vi "Barcode Print.vi"(1 "part type":string, 2 "Manual?":bool, 4 "error in":errorcluster, 5 "Part History Number":string, 6 "Plant Number":u8 max=9, 7 "Customer Number":string, 8 "Color":string, 9 "Serial Number":string, 10 "Inalfa Part Number":string, 11 "Frame Barcode Formats":T1[](array[typedef])) -> (0 "error out":errorcluster)   [LabVIEW 2018]
uses:
  typedefs/barcode format params.ctl
  typedefs/barcode printer types.ctl
  typedefs/open tcp connections.ctl
  <vilib>/Instr/_visa.llb/VISA Configure Serial Port (Instr).vi
panel:
  out "concatenated string":string
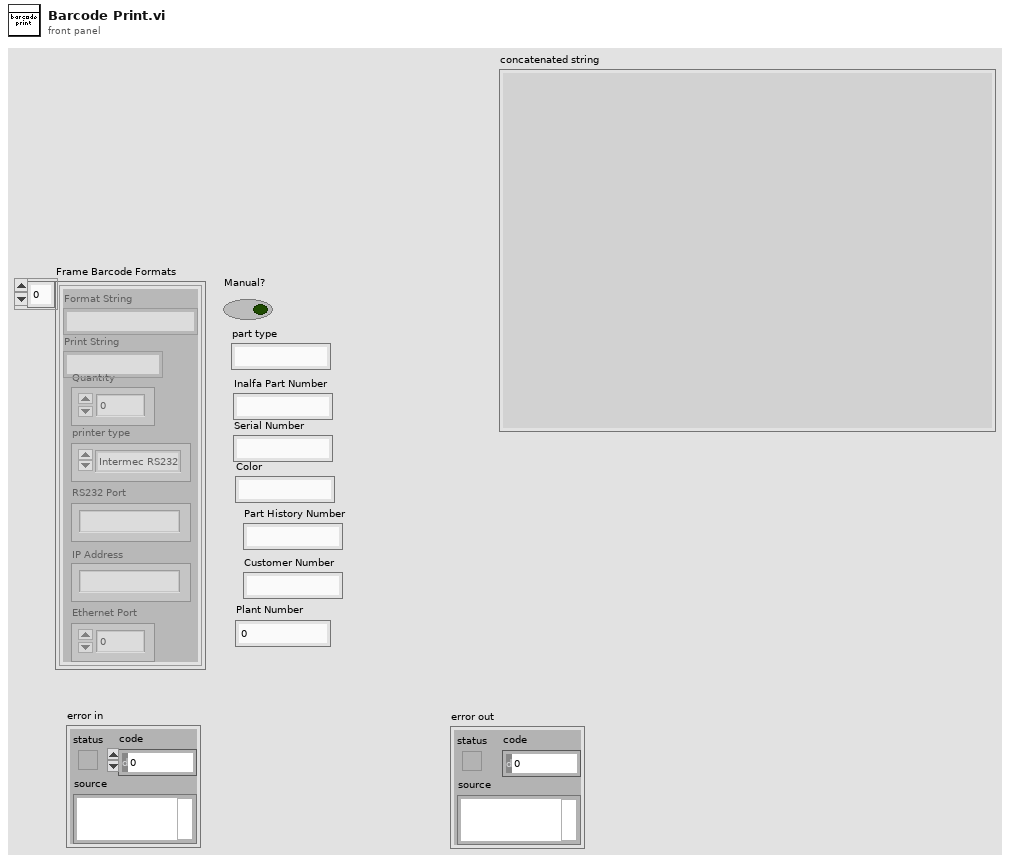
[diagram p1: front panel]
types:
  T1 = typedef "barcode format params.ctl" = cluster{"Format String":string, "Print String":string, "Quantity":u8, "printer type":T2, "RS232 Port":string, "IP Address":string, "Ethernet Port":u32}
  T2 = typedef "barcode printer types.ctl" = enum16{"Intermec RS232", "Intermec Ethernet"}
  T3 = typedef "open tcp connections.ctl" = cluster{"ip address":string, "connection ID":refnum<k5>}
  T4 = cluster{"Frame Barcode Formats":T1[], "VISA resource name":refnum<visa-resource-name>, "Format String":string, "Print String":string, "Inalfa Part Number":string, "Serial Number":string, "Color":string, "Customer Number":string, "Part History Number":string, "Plant Number":u8, "Manual?":bool, "part type":string, "to print":string[], "open rs232 ports":refnum<visa-resource-name>[], "open tcp ports":T3[]}
  T5 = typedef "imagedata.ctl" = cluster{"image type":i32, "image depth":i32, "image":u8[], "mask":u8[], "colors":u32[], "Rectangle":cluster{"left":i16, "top":i16, "right":i16, "bottom":i16}}
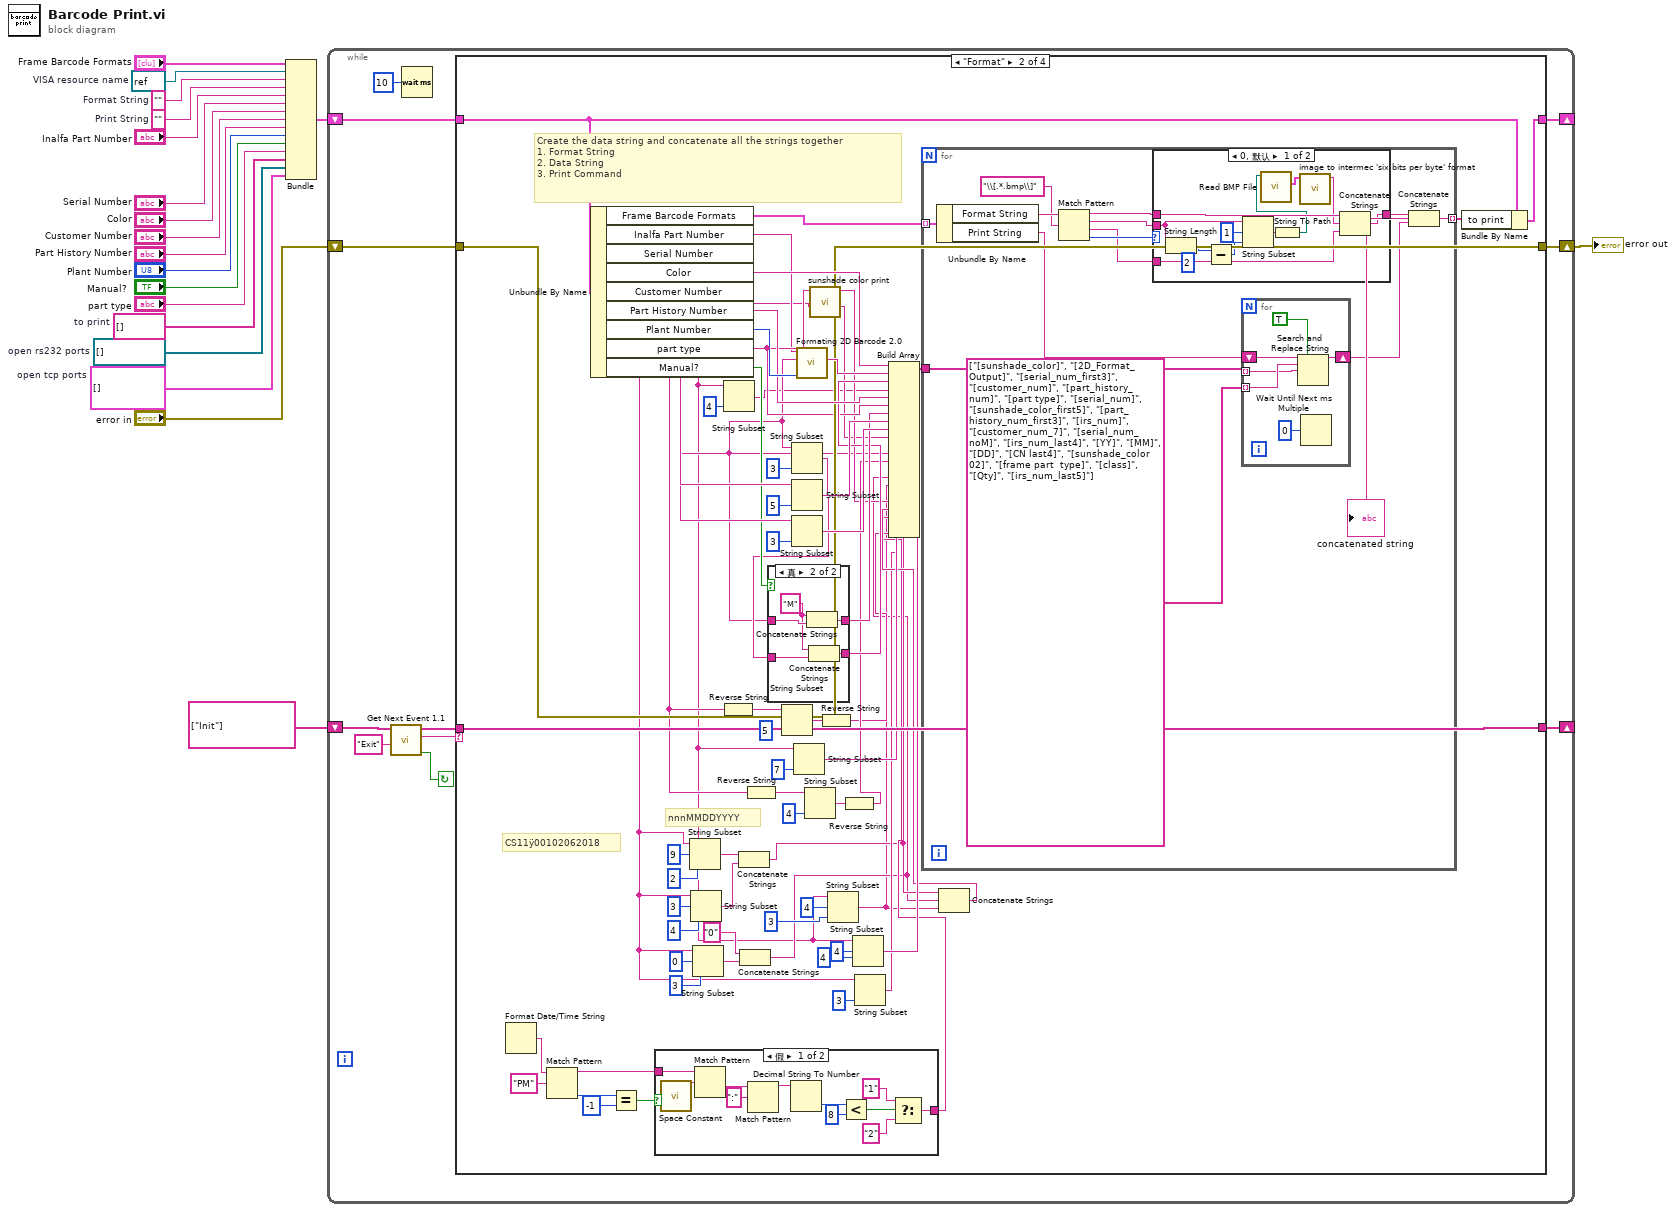
[diagram p0: block diagram]
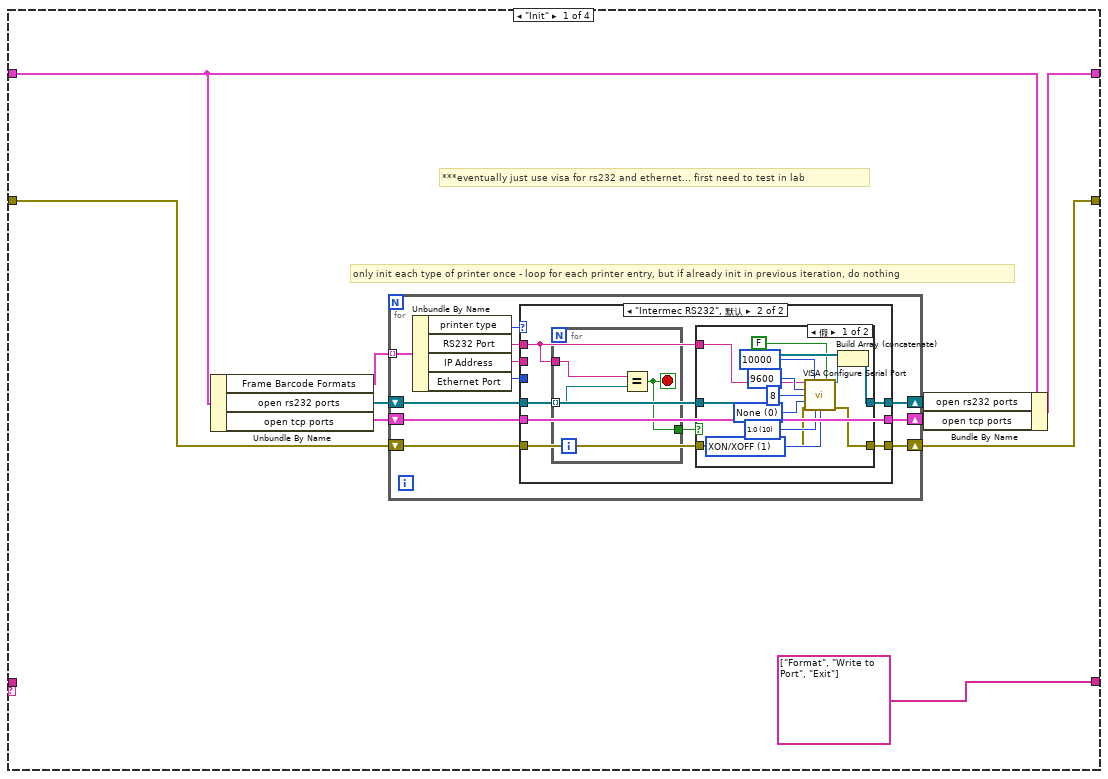
[diagram p2: hidden frame]
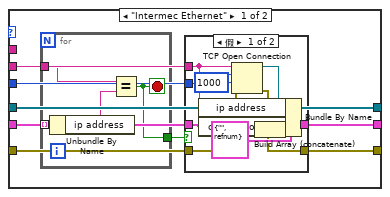
[diagram p3: hidden frame]
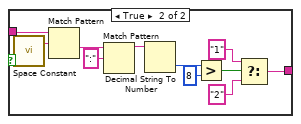
[diagram p6: hidden frame]
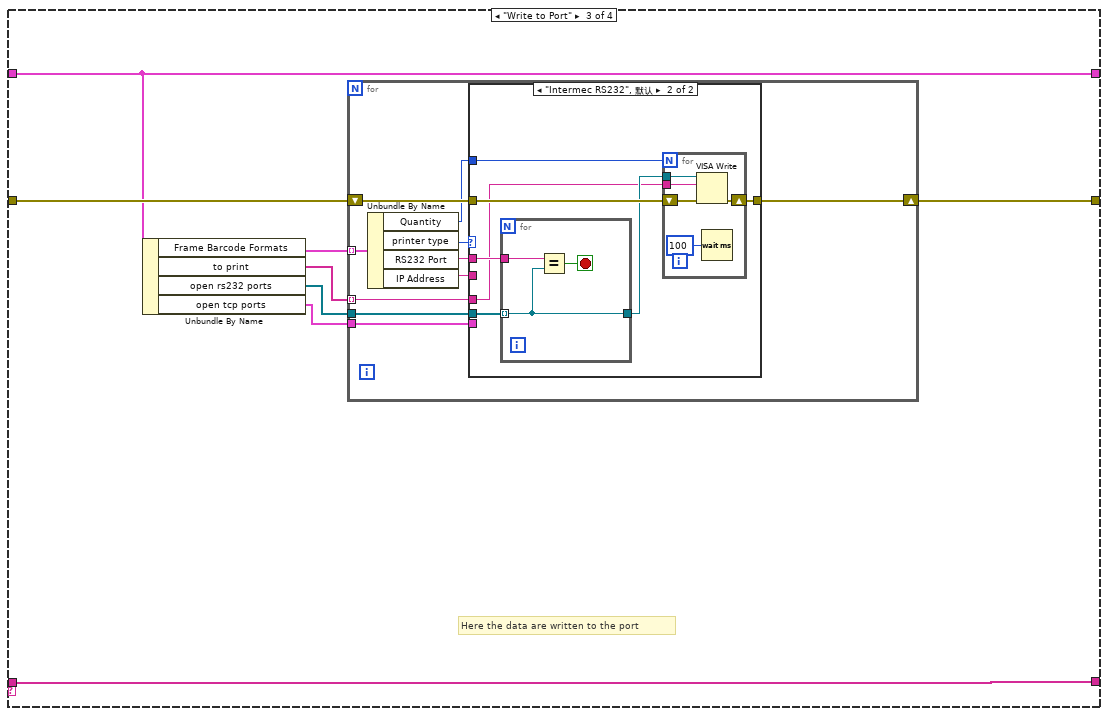
[diagram p9: hidden frame]
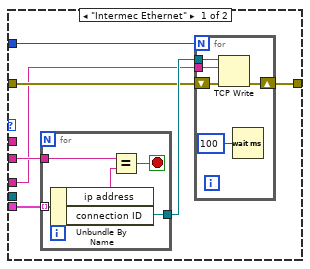
[diagram p10: hidden frame]
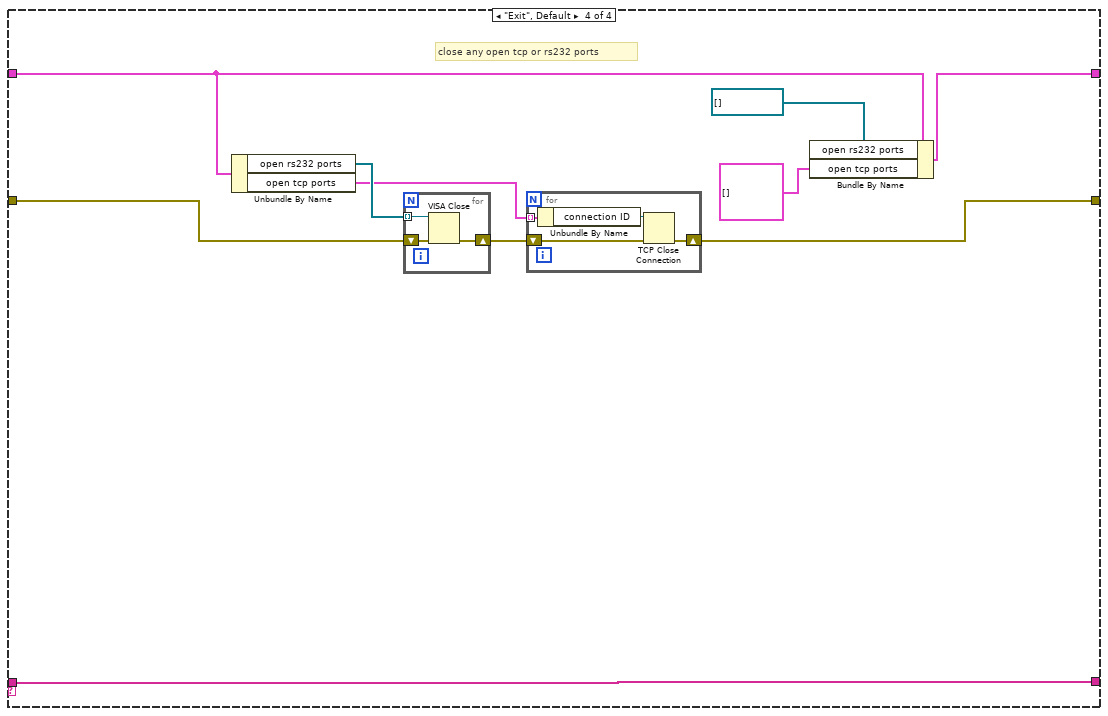
[diagram p11: hidden frame]
diagram:
  w1 = T3[] []  # open tcp ports
  w2 = refnum<visa-resource-name>[] []  # open rs232 ports
  w3 = string[] []  # to print
  w16 = ""  # Print String
  w17 = refnum<visa-resource-name> refnum  # VISA resource name
  w18 = ""  # Format String
  n1 = Bundle("Frame Barcode Formats"="Frame Barcode Formats", "VISA resource name"=w17, "Format String"=w18, "Print String"=w16, "Inalfa Part Number"="Inalfa Part Number", "Serial Number"="Serial Number", "Color"="Color", "Customer Number"="Customer Number", "Part History Number"="Part History Number", "Plant Number"="Plant Number", "Manual?"="Manual?", "part type"="part type", "to print"=w3, "open rs232 ports"=w2, "open tcp ports"=w1) -> (w19:T4)  [unwired: 1 in]
  n2 = while {
    shift-right: [w28] -> _
    shift-left: string[] ["Init"] ("Event queue out") -> [w27]
    shift-right: [w24] -> _
    shift-left: w19 -> [w25]
    shift-right: [w20] -> w4
    shift-left: "error in" -> [w21]
    stop <- w26 continue-if-true
    n3 = call "Get Next Event 1.1.vi"("Exit Event"="Exit", "event queue in"=w27) -> ("Condition (Exit:F)"=w26:bool, "next event"=w30:string, "event queue out"=w29:string[])  [unwired: 6 in, 1 out]
    n4 = Wait (ms)(milliseconds to wait=u32 10) -> ()  [unwired: 1 out]
    n5 = case shown="\"Format\"" w30 {
      tunnel: w29 -> [_ w148 w234 w286]
      tunnel: [string[] ["Format", "Write to Port", "Exit"] ("event queue out") w148 w234 w286] -> w28
      tunnel: w25 -> [w38 w166 w231 w281]
      tunnel: [w40 w165 w231 w280] -> w24
      tunnel: w21 -> [w35 w139 w233 w285]
      tunnel: [w34 w139 w232 w283] -> w20
      frame "Init" {
        # "***eventually just use visa for rs232 and ethernet... first need to test in lab"
        # "only init each type of printer once - loop for each printer entry, but if already init in previous iteration, do nothing"
        n6 = Unbundle By Name(w38) -> ("Frame Barcode Formats"=w33:T1[], "open rs232 ports"=w32:refnum<visa-resource-name>[], "open tcp ports"=w31:T3[])
        n7 = for {
          tunnel: w33 -> [w51] mode=indexing
          shift-right: [w45] -> w37
          shift-left: w32 -> [w47]
          shift-right: [w46] -> w36
          shift-left: w31 -> [w48]
          shift-right: [w41] -> w34
          shift-left: w35 -> [w49]
          n8 = Unbundle By Name(w51) -> ("printer type"=w50:T2, "RS232 Port"=w44:string, "IP Address"=w43:string, "Ethernet Port"=w42:u32)
          n9 = case shown="\"Intermec RS232\", 默认" w50 {
            tunnel: w49 -> [w53 w77]
            tunnel: w48 -> [w56 w81]
            tunnel: w47 -> [w59 w80]
            tunnel: [w57 w81] -> w46
            tunnel: [w59 w79] -> w45
            tunnel: w44 -> [_ w78]
            tunnel: w43 -> [w55 _]
            tunnel: w42 -> [w54 _]
            tunnel: [w52 w76] -> w41
            frame "Intermec Ethernet" {
              n10 = for {
                tunnel: w56 -> [w75] mode=indexing
                tunnel: w55 -> [w74]
                tunnel: [w72] -> w58
                stop <- w72 stop-if-true
                n11 = Unbundle By Name(w75) -> ("ip address"=w73:string)
                n12 = Equal?(x=w74, y=w73) -> (x = y?=w72:bool)
              }
              n13 = case shown="假" w58 {
                tunnel: [w66 w71] -> w57
                tunnel: w56 -> [w67 w71]
                tunnel: w55 -> [w63 _]
                tunnel: w54 -> [w69 _]
                tunnel: w53 -> [w61 w70]
                tunnel: [w60 w70] -> w52
                frame False {
                  n14 = TCP Open Connection(address=w63, remote port or service name=w69, timeout ms (60000)=1000, error in (no error)=w61) -> (connection ID=w62:refnum<k5>, error out=w60:errorcluster)  [unwired: 1 in]
                  n15 = Bundle By Name(cluster=T3 {"ip address"="", "connection ID"=refnum}, "ip address"=w63, "connection ID"=w62) -> (w64:T3)
                  n16 = Build Array (concatenate)(w67, w64) -> (w66:T3[])
                }
                frame True {
                }
              }
            }
            frame "Intermec RS232", Default {
              n17 = for {
                tunnel: w80 -> [w98] mode=indexing
                tunnel: w78 -> [w100]
                tunnel: [w99] -> w82
                stop <- w99 stop-if-true
                n18 = Equal?(x=w100, y=w98) -> (x = y?=w99:bool)
              }
              n19 = case shown="假" w82 {
                tunnel: w80 -> [w95 w97]
                tunnel: [w94 w97] -> w79
                tunnel: w78 -> [w86 _]
                tunnel: w77 -> [w84 w96]
                tunnel: [w83 w96] -> w76
                frame False {
                  w88 = u16 1 items=["None"=0, "XON/XOFF"=1, "RTS/CTS"=2, "DTR/DSR"=4] ("flow control")
                  w89 = u16 10 items=["1.0"=10, "1.5"=15, "2.0"=20] ("stop bits")
                  w92 = u16 0 items=["None", "Odd", "Even", "Mark", "Space"] ("parity")
                  n20 = call-poly "VISA Configure Serial Port"("VISA resource name"=w86, "timeout (10sec)"=u32 10000, "Enable Termination\nChar (T)"=FALSE ("Enable Termination Char (T)"), "baud rate (9600)"=u32 9600 ("baud rate"), "data bits (8)"=u16 8 ("data bits"), "parity (0:none)"=w92, "error in (no error)"=w84, "stop bits (10: 1 bit)"=w89, "flow control (0:none)"=w88) -> ("VISA resource name out"=w85:refnum<visa-resource-name>, "error out"=w83:errorcluster)  [unwired: 5 in]
                  n21 = Build Array (concatenate)(w95, w85) -> (w94:refnum<visa-resource-name>[])
                }
                frame True {
                }
              }
            }
          }
        }
        n22 = Bundle By Name(cluster=w38, "open rs232 ports"=w37, "open tcp ports"=w36) -> (w40:T4)
      }
      frame "Format" {
        # "CS11ÿ00102062018"
        # "nnnMMDDYYYY"
        # "Create the data string and concatenate all the strings together\n1. Format String\n2. Data String\n3. Print Command"
        n23 = Format Date/Time String() -> (date/time string=w130:string)  [unwired: 3 in]
        n24 = Match Pattern(string=w130, regular expression="PM") -> (before substring=w125:string, offset past match=w128:i32)  [unwired: 1 in, 2 out]
        n25 = Unbundle By Name(w166) -> ("Frame Barcode Formats"=w164:T1[], "Inalfa Part Number"=w120:string, "Serial Number"=w110:string, "Color"=w154:string, "Customer Number"=w102:string, "Part History Number"=w153:string, "Plant Number"=w160:u8, "part type"=w135:string, "Manual?"=w152:bool)
        n26 = Equal?(x=w128, y=-1) -> (x = y?=w126:bool)
        n27 = case shown="假" w126 {
          tunnel: w125 -> [w169 w188]
          tunnel: [w168 w179] -> w124
          frame False {
            n28 = call <vilib>:"Space Constant.vi"() -> ("String"=w177:string)
            n29 = Match Pattern(string=w169, regular expression=w177) -> (after substring=w176:string)  [unwired: 1 in, 3 out]
            n30 = Match Pattern(string=w176, regular expression=":") -> (before substring=w167:string)  [unwired: 1 in, 3 out]
            n31 = Decimal String To Number(string=w167) -> (number=w174:i32)  [unwired: 2 in, 1 out]
            n32 = Less?(x=w174, y=8) -> (x < y?=w172:bool)
            n33 = Select(t="1" ("regular expression"), s=w172, f="2" ("regular expression")) -> (s? t:f=w168:string)
          }
          frame True {
            n34 = call <vilib>:"Space Constant.vi"() -> ("String"=w187:string)
            n35 = Match Pattern(string=w188, regular expression=w187) -> (after substring=w186:string)  [unwired: 1 in, 3 out]
            n36 = Match Pattern(string=w186, regular expression=":") -> (before substring=w178:string)  [unwired: 1 in, 3 out]
            n37 = Decimal String To Number(string=w178) -> (number=w184:i32)  [unwired: 2 in, 1 out]
            n38 = Greater?(x=w184, y=8) -> (0:w182:bool)
            n39 = Select(t="1" ("regular expression"), s=w182, f="2" ("regular expression")) -> (s? t:f=w179:string)
          }
        }
        n40 = String Subset(string=w110, offset (0)=9, length (rest)=2 ("length (rest)")) -> (substring=w114:string)
        n41 = String Subset(string=w110, offset (0)=3, length (rest)=4 ("length (rest)")) -> (substring=w113:string)
        n42 = String Subset(string=w110, offset (0)=0, length (rest)=3 ("length (rest)")) -> (substring=w107:string)
        n43 = Reverse String(1:w120) -> (0:w123:string)
        n44 = String Subset(string=w102, length (rest)=4 ("length (rest)")) -> (substring=w103:string)  [unwired: 1 in]
        n45 = Concatenate Strings(w114, w113) -> (w109:string)
        n46 = Concatenate Strings("0" ("string"), w107) -> (w106:string)
        n47 = Reverse String(1:w120) -> (0:w143:string)
        n48 = String Subset(string=w123, length (rest)=5 ("length (rest)")) -> (substring=w122:string)  [unwired: 1 in]
        n49 = String Subset(string=w110, length (rest)=3 ("length (rest)")) -> (substring=w150:string)  [unwired: 1 in]
        n50 = case shown="真" w152 {
          tunnel: w110 -> [w190 w195]
          tunnel: [w190 w194] -> w151
          tunnel: w150 -> [w189 w193]
          tunnel: [w189 w191] -> w149
          frame False {
          }
          frame True {
            w192 = "M" ("string")
            n51 = Concatenate Strings(w192, w195) -> (w194:string)
            n52 = Concatenate Strings(w192, w193) -> (w191:string)
          }
        }
        n53 = String Subset(string=w154, length (rest)=5 ("length (rest)")) -> (substring=w156:string)  [unwired: 1 in]
        n54 = String Subset(string=w153, length (rest)=3 ("length (rest)")) -> (substring=w155:string)  [unwired: 1 in]
        n55 = String Subset(string=w102, length (rest)=7 ("length (rest)")) -> (substring=w146:string)  [unwired: 1 in]
        n56 = call "Formating 2D Barcode 2.0.vi"("Plant Number"=w160, "Serial Number"=w110, "IRS Number"=w120) -> ("2-D Barcode"=w159:string)  [unwired: 8 in]
        n57 = String Subset(string=w143, length (rest)=4 ("length (rest)")) -> (substring=w145:string)  [unwired: 1 in]
        n58 = call "sunshade color print.vi"("custom number"=w102, "part type"=w135) -> ("Inalfa Part Number"=w105:string, "sunshade color"=w134:string)  [unwired: 8 in]
        n59 = Reverse String(1:w122) -> (0:w121:string)
        n60 = String Subset(string=w102, offset (0)=4, length (rest)=3 ("length (rest)")) -> (substring=w101:string)
        n61 = Reverse String(1:w145) -> (0:w142:string)
        n62 = String Subset(string=w102, offset (0)=4, length (rest)=4 ("length (rest)")) -> (substring=w136:string)
        n63 = String Subset(string=w110, length (rest)=3 ("length (rest)")) -> (substring=w131:string)  [unwired: 1 in]
        n64 = Concatenate Strings(w109, w106, w101) -> (w133:string)
        n65 = Build Array(w154, w159, w149, w103, w153, w135, w151, w156, w155, w105, w146, w110, w142, w109, w106, w101, w136, w134, w133, w124, w131, w121) -> (w162:string[])
        n66 = for {
          tunnel: w164 -> [w207] mode=indexing
          tunnel: [w208] -> w163 mode=indexing
          tunnel: w162 -> [w204]
          n67 = Unbundle By Name(w207) -> ("Format String"=w201:string, "Print String"=w206:string)
          n68 = Match Pattern(string=w201, regular expression="\\[.*.bmp\\]" ("search string/char (-)")) -> (before substring=w198:string, match substring=w196:string, after substring=w197:string, offset past match=w199:i32)  [unwired: 1 in]
          n69 = case shown="0, 默认" w199 {
            tunnel: [w219 w221] -> w202
            tunnel: w198 -> [w220 w221]
            tunnel: w196 -> [w214 _]
            tunnel: w197 -> [w215 _]
            frame 0, Default {
              n70 = String Length(string=w214) -> (length=w212:i32)
              n71 = Subtract(x=w212, y=2) -> (x-y=w210:i32)
              n72 = String Subset(string=w214, offset (0)=1, length (rest)=w210) -> (substring=w209:string)
              n73 = String To Path(string=w209) -> (path=w217:path)
              n74 = call <vilib>:"Read BMP File.vi"("path to BMP file"=w217) -> ("image data"=w218:T5)  [unwired: 8 in, 2 out]
              n75 = call "image to intermec 'six bits per byte' format.vi"("image data"=w218) -> ("six bits per byte"=w216:string)  [unwired: 10 in]
              n76 = Concatenate Strings(w220, w216, w215) -> (w219:string)
            }
            frame ..-1 {
            }
          }
          n77 = for {
            shift-right: [w225] -> w203
            shift-left: w206 -> [w226]
            tunnel: string[] ["[sunshade_color]", "[2D_Format_Output]", "[serial_num_first3]", "[customer_num]", "[part_history_num]", "[part type]", "[serial_num]", "[sunshade_color_first5]", "[part_history_num_first3]", "[irs_num]", "[customer_num_7]", "[serial_num_noM]", "[irs_num_last4]", "[YY]", "[MM]", "[DD]", "[CN last4]", "[sunshade_color 02]", "[frame part  type]", "[class]", "[Qty]", "[irs_num_last5]"] -> [w224] mode=indexing
            tunnel: w204 -> [w223] mode=indexing
            n78 = Search and Replace String(replace all?=TRUE ("replace all? (F)"), input string=w226, search string=w224, replace string=w223) -> (result string=w225:string)  [unwired: 4 in, 3 out]
            n79 = Wait Until Next ms Multiple(millisecond multiple=u32 0) -> ()  [unwired: 1 out]
          }
          n80 = Concatenate Strings(w202, w203) -> (w208:string)
          "concatenated string" <- w208
        }
        n81 = Bundle By Name(cluster=w166, "to print"=w163) -> (w165:T4)
      }
      frame "Write to Port" {
        # "Here the data are written to the port"
        n82 = Unbundle By Name(w231) -> ("Frame Barcode Formats"=w235:T1[], "to print"=w230:string[], "open rs232 ports"=w229:refnum<visa-resource-name>[], "open tcp ports"=w228:T3[])
        n83 = for {
          shift-right: [w243] -> w232
          shift-left: w233 -> [w244]
          tunnel: w235 -> [w245] mode=indexing
          tunnel: w230 -> [w239] mode=indexing
          tunnel: w229 -> [w241]
          tunnel: w228 -> [w240]
          n84 = Unbundle By Name(w245) -> ("Quantity"=w236:u8, "printer type"=w238:T2, "RS232 Port"=w242:string, "IP Address"=w237:string)
          n85 = case shown="\"Intermec RS232\", 默认" w238 {
            tunnel: w240 -> [w252 _]
            tunnel: w241 -> [_ w269]
            tunnel: w242 -> [_ w268]
            tunnel: w237 -> [w251 _]
            tunnel: w244 -> [w249 w267]
            tunnel: [w248 w266] -> w243
            tunnel: w239 -> [w247 w264]
            tunnel: w236 -> [w246 w263]
            frame "Intermec Ethernet" {
              n86 = for {
                tunnel: w252 -> [w262] mode=indexing
                tunnel: w251 -> [w261]
                tunnel: [w258] -> w250
                stop <- w259 stop-if-true
                n87 = Unbundle By Name(w262) -> ("ip address"=w260:string, "connection ID"=w258:refnum<k5>)
                n88 = Equal?(x=w261, y=w260) -> (x = y?=w259:bool)
              }
              n89 = for {
                N: w246 -> [_]
                tunnel: w250 -> [w257]
                tunnel: w247 -> [w254]
                shift-right: [w255] -> w248
                shift-left: w249 -> [w256]
                n90 = TCP Write(connection ID=w257, data in=w254, error in (no error)=w256) -> (error out=w255:errorcluster)  [unwired: 1 in, 2 out]
                n91 = Wait (ms)(milliseconds to wait=u32 100) -> ()  [unwired: 1 out]
              }
            }
            frame "Intermec RS232", Default {
              n92 = for {
                tunnel: w269 -> [w275] mode=indexing
                tunnel: w268 -> [w277]
                tunnel: [w275] -> w265
                stop <- w276 stop-if-true
                n93 = Equal?(x=w277, y=w275) -> (x = y?=w276:bool)
              }
              n94 = for {
                N: w263 -> [_]
                tunnel: w265 -> [w272]
                tunnel: w264 -> [w271]
                shift-right: [w273] -> w266
                shift-left: w267 -> [w274]
                n95 = VISA Write(VISA resource name=w272, write buffer=w271, error in (no error)=w274) -> (error out=w273:errorcluster)  [unwired: 2 out]
                n96 = Wait (ms)(milliseconds to wait=u32 100) -> ()  [unwired: 1 out]
              }
            }
          }
        }
      }
      frame "Exit", Default {
        # "close any open tcp or rs232 ports"
        n97 = Unbundle By Name(w281) -> ("open rs232 ports"=w287:refnum<visa-resource-name>[], "open tcp ports"=w282:T3[])
        n98 = for {
          tunnel: w287 -> [w294] mode=indexing
          shift-right: [w292] -> w284
          shift-left: w285 -> [w293]
          n99 = VISA Close(VISA resource name=w294, error in (no error)=w293) -> (error out=w292:errorcluster)
        }
        n100 = for {
          shift-right: [w290] -> w283
          shift-left: w284 -> [w291]
          tunnel: w282 -> [w289] mode=indexing
          n101 = Unbundle By Name(w289) -> ("connection ID"=w288:refnum<k5>)
          n102 = TCP Close Connection(connection ID=w288, error in (no error)=w291) -> (error out=w290:errorcluster)  [unwired: 1 in, 1 out]
        }
        n103 = Bundle By Name(cluster=w281, "open rs232 ports"=refnum<visa-resource-name>[] [], "open tcp ports"=T3[] []) -> (w280:T4)
      }
    }
  }
  "error out" <- w4
